vi "Create Listener.vi"(8 "error in (no error)":errorcluster, 11 "TCP slave in":refnum<class "TCP Slave.lvclass">) -> (0 "error out":errorcluster, 3 "TCP slave out":refnum<class "TCP Slave.lvclass">)   [LabVIEW 2015, in "SubVIs.lvlib" / "TCP Slave.lvclass"]
doc: "Creates a new listener on the stored port, and then stores that in the class."
uses:
  <vilib>/Modbus/subvis/Protocol/TCP/TCP Slave/TCP Slave.lvclass
  <vilib>/Modbus/subvis/Protocol/TCP/TCP Slave/TCP Slave.lvclass/TCP Slave.ctl
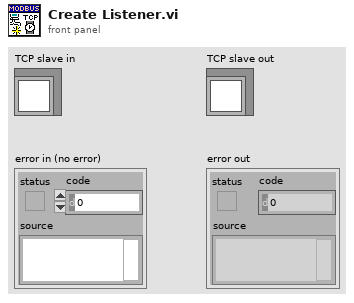
[diagram p1: front panel]
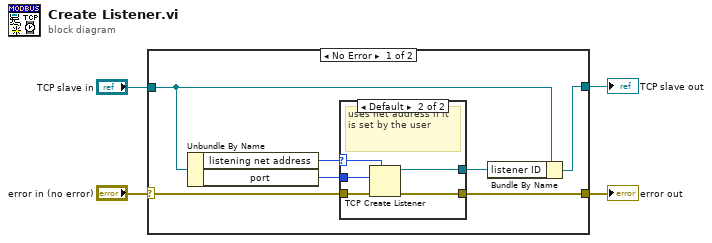
[diagram p0: block diagram]
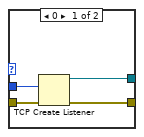
[diagram p2: hidden frame]
diagram:
  n1 = case shown="No Error" "error in (no error)" {
    selector: "error in (no error)" -> [w5 w21]
    tunnel: [w11 w21] -> w4
    tunnel: "TCP slave in" -> [w10 w22]
    tunnel: [w9 w22] -> w2
    frame No Error {
      n2 = Unbundle By Name(w10) -> ("listening net address"=w6:u32, "port"=w8:u16)
      n3 = case shown="Default" w6 {
        selector: w6 -> [_ w16]
        tunnel: w5 -> [w15 w20]
        tunnel: [w13 w19] -> w11
        tunnel: w8 -> [w14 w18]
        tunnel: [w12 w17] -> w7
        frame 0 {
          n4 = TCP Create Listener(8:w15, 10:w14) -> (0:w13:errorcluster, 3:w12:refnum<k5>)  [unwired: 3 in, 1 out]
        }
        frame Default {
          # "uses net address if it is set by the user"
          n5 = TCP Create Listener(7:w16, 8:w20, 10:w18) -> (0:w19:errorcluster, 3:w17:refnum<k5>)  [unwired: 2 in, 1 out]
        }
      }
      n6 = Bundle By Name(cluster=w10, "listener ID"=w7) -> (w9:refnum<class "TCP Slave.lvclass">)
    }
    frame Error {
    }
  }
  "error out" <- w4
  "TCP slave out" <- w2
